vi "OCV Histogram gRPC.vi"() -> (1 "mean values of channels":dbl[](array[numeric]), 2 "std dev":dbl, 3 "range":dbl)   [LabVIEW 2019] (continued)
  out "Waveform Chart ch0":sgl[](graph)=[3.4816353, 3.4816356, 3.4816363, 3.4816382, 3.4816408, 3.48164, 3.481639, 3.4816341, 3.481641, 3.4816356, 3.4816346, 3.4816375, 3.4816372, 3.481637, 3.4816399, 3.4816375, 3.4816432, 3.4816358, 3.4816375, 3.48164, 3.4816394, 3.4816341, 3.4816387, 3.4816349, 3.4816382, 3.481638, 3.4816375, 3.4816344, 3.4816382, 3.4816399, 3.4816442, 3.4816413, 3.481636, 3.4816372, 3.4816327, 3.4816341, 3.4816403, 3.4816394, 3.4816413, 3.4816415, 3.4816406, 3.481637, 3.4816372, 3.4816396, 3.4816391, 3.481643, 3.4816375, 3.4816341, 3.4816446, 3.4816337, 3.4816325, 3.4816356, 3.4816365, 3.4816322, 3.4816391, 3.481637, 3.4816382, 3.4816358, 3.4816394, 3.481634, 3.4816377, 3.481638, 3.4816375, 3.4816403, 3.4816413, 3.4816382, 3.481636, 3.4816418, 3.4816382, 3.4816322, 3.4816375, 3.4816356, 3.481642, 3.4816384, 3.4816382, 3.4816365, 3.481637, 3.4816353, 3.4816394, 3.4816382, 3.4816437, 3.4816415, 3.4816375, 3.4816375, 3.4816418, 3.4816406, 3.4816408, 3.4816415, 3.4816391, 3.4816394, 3.4816334, 3.48164, 3.4816394, 3.481636, 3.4816372, 3.4816384, 3.4816353, 3.4816396, 3.4816408, 3.481637, 3.4816346, 3.4816408, 3.4816375, 3.4816356, 3.481638, 3.4816396, 3.4816358, 3.4816408, 3.4816396, 3.4816313, 3.481634, 3.4816365, 3.481638, 3.4816403, 3.4816394, 3.4816377, 3.4816372, 3.4816365, 3.4816365, 3.4816382, 3.481635, 3.481638, 3.481636, 3.4816415, 3.481636, 3.4816332, 3.4816341, 3.4816382, 3.4816413, 3.4816377, 3.4816337, 3.4816344, 3.4816356, 3.4816418, 3.4816408, 3.4816337, 3.4816363, 3.481636, 3.481641, 3.4816375, 3.4816408, 3.4816346, 3.4816341, 3.4816403, 3.4816408, 3.4816437, 3.4816349, 3.481637, 3.4816344, 3.481637, 3.4816344, 3.4816406, 3.4816418, 3.481639, 3.481636, 3.4816332, 3.481638, 3.4816372, 3.481633, 3.4816353, 3.4816415, 3.4816365, 3.481645, 3.4816349, 3.481638, 3.4816444, 3.481642, 3.4816356, 3.481642, 3.4816377, 3.4816396, 3.4816408, 3.4816327, 3.4816408, 3.4816368, 3.481637, 3.4816332, 3.481636, 3.481638, 3.4816399, 3.4816365, 3.4816375, 3.4816287, 3.481641, 3.4816341, 3.4816413, 3.4816396, 3.4816425, 3.4816406, 3.481635, 3.4816413, 3.4816387, 3.4816396, 3.4816391, 3.4816377, 3.4816406, 3.481641, 3.4816406, 3.481635, 3.4816337]
  out "Waveform Chart ch3":sgl[](graph)=[3.482367, 3.4823706, 3.4823644, 3.4823663, 3.48237, 3.4823658, 3.482369, 3.4823651, 3.482372, 3.4823728, 3.4823637, 3.4823651, 3.4823728, 3.482369, 3.4823713, 3.4823675, 3.482368, 3.4823685, 3.4823701, 3.4823718, 3.4823713, 3.4823737, 3.482368, 3.482367, 3.4823716, 3.4823666, 3.482369, 3.4823692, 3.4823682, 3.482368, 3.482372, 3.482368, 3.482369, 3.4823658, 3.48237, 3.4823718, 3.482369, 3.4823678, 3.482369, 3.4823713, 3.4823692, 3.4823666, 3.4823666, 3.4823713, 3.482368, 3.482366, 3.482367, 3.48237, 3.4823694, 3.4823694, 3.4823673, 3.482366, 3.4823682, 3.4823666, 3.4823685, 3.482366, 3.48237, 3.4823682, 3.4823692, 3.4823651, 3.482369, 3.48237, 3.4823647, 3.4823694, 3.482367, 3.4823701, 3.482367, 3.482368, 3.4823678, 3.4823651, 3.4823635, 3.482366, 3.482366, 3.4823685, 3.4823694, 3.4823656, 3.4823709, 3.4823658, 3.4823673, 3.4823682, 3.4823694, 3.482367, 3.482367, 3.4823663, 3.4823596, 3.4823644, 3.4823697, 3.4823694, 3.482368, 3.4823668, 3.4823647, 3.4823644, 3.482364, 3.4823663, 3.4823635, 3.4823613, 3.482367, 3.4823625, 3.4823687, 3.482369, 3.4823632, 3.4823682, 3.4823718, 3.4823654, 3.48237, 3.482371, 3.4823675, 3.4823616, 3.4823694, 3.482364, 3.4823709, 3.4823658, 3.4823692, 3.4823651, 3.4823654, 3.4823618, 3.4823678, 3.4823644, 3.4823694, 3.4823668, 3.482365, 3.4823606, 3.4823675, 3.4823725, 3.4823642, 3.4823651, 3.4823678, 3.4823651, 3.4823666, 3.4823637, 3.4823608, 3.4823682, 3.4823635, 3.4823654, 3.4823651, 3.4823635, 3.482366, 3.482362, 3.4823654, 3.4823697, 3.4823678, 3.482368, 3.4823656, 3.4823704, 3.4823687, 3.482368, 3.4823687, 3.4823644, 3.4823673, 3.4823682, 3.48237, 3.4823701, 3.4823663, 3.4823632, 3.482362, 3.4823678, 3.4823663, 3.482365, 3.4823642, 3.4823697, 3.4823642, 3.4823658, 3.4823675, 3.482364, 3.4823694, 3.4823692, 3.482372, 3.482364, 3.4823654, 3.4823654, 3.4823637, 3.482367, 3.4823623, 3.482365, 3.4823625, 3.4823656, 3.482365, 3.4823658, 3.4823635, 3.4823668, 3.4823666, 3.482368, 3.4823678, 3.482362, 3.4823651, 3.4823654, 3.4823692, 3.4823673, 3.4823668, 3.4823666, 3.482364, 3.4823673, 3.4823701, 3.4823651, 3.4823647, 3.4823635, 3.4823675, 3.4823632, 3.4823704, 3.4823666]
  out "Results Cluster":T4={"Waveform Chart ch0"=[3.481635332107544, 3.481635570526123, 3.4816362857818604, 3.481638193130493, 3.4816408157348633, 3.481640100479126, 3.4816389083862305, 3.4816341400146484, 3.4816410541534424, 3.481635570526123, 3.4816346168518066, 3.481637477874756, 3.4816372394561768, 3.4816370010375977, 3.481639862060547, 3.481637477874756, 3.4816431999206543, 3.481635808944702, 3.481637477874756, 3.481640100479126, 3.4816393852233887, 3.4816341400146484, 3.4816386699676514, 3.4816348552703857, 3.481638193130493, 3.481637954711914, 3.481637477874756, 3.4816343784332275, 3.481638193130493, 3.481639862060547, 3.4816441535949707, 3.4816412925720215, 3.4816360473632812, 3.4816372394561768, 3.481632709503174, 3.4816341400146484, 3.481640338897705, 3.4816393852233887, 3.4816412925720215, 3.4816415309906006, 3.481640577316284, 3.4816370010375977, 3.4816372394561768, 3.4816396236419678, 3.4816391468048096, 3.481642961502075, 3.481637477874756, 3.4816341400146484, 3.481644630432129, 3.4816336631774902, 3.4816324710845947, 3.481635570526123, 3.4816365242004395, 3.4816322326660156, 3.4816391468048096, 3.4816370010375977, 3.481638193130493, 3.481635808944702, 3.4816393852233887, 3.4816339015960693, 3.481637716293335, 3.481637954711914, 3.481637477874756, 3.481640338897705, 3.4816412925720215, 3.481638193130493, 3.4816360473632812, 3.4816417694091797, 3.481638193130493, 3.4816322326660156, 3.481637477874756, 3.481635570526123, 3.481642007827759, 3.4816384315490723, 3.481638193130493, 3.4816365242004395, 3.4816370010375977, 3.481635332107544, 3.4816393852233887, 3.481638193130493, 3.4816436767578125, 3.4816415309906006, 3.481637477874756, 3.481637477874756, 3.4816417694091797, 3.481640577316284, 3.4816408157348633, 3.4816415309906006, 3.4816391468048096, 3.4816393852233887, 3.481633424758911, 3.481640100479126, 3.4816393852233887, 3.4816360473632812, 3.4816372394561768, 3.4816384315490723, 3.481635332107544, 3.4816396236419678, 3.4816408157348633, 3.4816370010375977, 3.4816346168518066, 3.4816408157348633, 3.481637477874756, 3.481635570526123, 3.481637954711914, 3.4816396236419678, 3.481635808944702, 3.4816408157348633, 3.4816396236419678, 3.481631278991699, 3.4816339015960693, 3.4816365242004395, 3.481637954711914, 3.481640338897705, 3.4816393852233887, 3.481637716293335, 3.4816372394561768, 3.4816365242004395, 3.4816365242004395, 3.481638193130493, 3.481635093688965, 3.481637954711914, 3.4816360473632812, 3.4816415309906006, 3.4816360473632812, 3.481633186340332, 3.4816341400146484, 3.481638193130493, 3.4816412925720215, 3.481637716293335, 3.4816336631774902, 3.4816343784332275, 3.481635570526123, 3.4816417694091797, 3.4816408157348633, 3.4816336631774902, 3.4816362857818604, 3.4816360473632812, 3.4816410541534424, 3.481637477874756, 3.4816408157348633, 3.4816346168518066, 3.4816341400146484, 3.481640338897705, 3.4816408157348633, 3.4816436767578125, 3.4816348552703857, 3.4816370010375977, 3.4816343784332275, 3.4816370010375977, 3.4816343784332275, 3.481640577316284, 3.4816417694091797, 3.4816389083862305, 3.4816360473632812, 3.481633186340332, 3.481637954711914, 3.4816372394561768, 3.481632947921753, 3.481635332107544, 3.4816415309906006, 3.4816365242004395, 3.481645107269287, 3.4816348552703857, 3.481637954711914, 3.48164439201355, 3.481642007827759, 3.481635570526123, 3.481642007827759, 3.481637716293335, 3.4816396236419678, 3.4816408157348633, 3.481632709503174, 3.4816408157348633, 3.4816367626190186, 3.4816370010375977, 3.481633186340332, 3.4816360473632812, 3.481637954711914, 3.481639862060547, 3.4816365242004395, 3.481637477874756, 3.481628656387329, 3.4816410541534424, 3.4816341400146484, 3.4816412925720215, 3.4816396236419678, 3.481642484664917, 3.481640577316284, 3.481635093688965, 3.4816412925720215, 3.4816386699676514, 3.4816396236419678, 3.4816391468048096, 3.481637716293335, 3.481640577316284, 3.4816410541534424, 3.481640577316284, 3.481635093688965, 3.4816336631774902], "ch0 mean"=3.4816378843784332, "ch0 range"=1.6450881958007812e-05, "ch0 std dev"=2.907318571584298e-06, "Histogram Graph ch0"={"X Values"=[3.481629478931427, 3.4816311240196227, 3.4816327691078186, 3.4816344141960145, 3.4816360592842104, 3.4816377043724063, 3.481639349460602, 3.481640994548798, 3.481642639636994, 3.48164428472519], "Histogram: h(x)"=[1, 1, 10, 26, 32, 51, 28, 39, 6, 6]}, "Waveform Chart ch1"=[3.4830455780029297, 3.483036756515503, 3.4830386638641357, 3.483046770095825, 3.483046531677246, 3.4830381870269775, 3.483044385910034, 3.4830410480499268, 3.483041763305664, 3.483039617538452, 3.483038902282715, 3.4830398559570312, 3.483046293258667, 3.483041286468506, 3.4830386638641357, 3.4830422401428223, 3.4830386638641357, 3.4830429553985596, 3.4830410480499268, 3.483044385910034, 3.4830453395843506, 3.483041286468506, 3.4830446243286133, 3.4830400943756104, 3.4830410480499268, 3.4830427169799805, 3.483039617538452, 3.4830408096313477, 3.4830451011657715, 3.4830451011657715, 3.483037233352661, 3.483043670654297, 3.483041763305664, 3.4830408096313477, 3.4830405712127686, 3.4830384254455566, 3.483039379119873, 3.4830453395843506, 3.483045816421509, 3.483043670654297, 3.4830434322357178, 3.4830405712127686, 3.4830427169799805, 3.483043909072876, 3.4830427169799805, 3.4830446243286133, 3.4830431938171387, 3.483044385910034, 3.4830422401428223, 3.483038902282715, 3.483041286468506, 3.483046054840088, 3.483045816421509, 3.483044385910034, 3.483041286468506, 3.4830398559570312, 3.4830427169799805, 3.4830434322357178, 3.483043909072876, 3.4830408096313477, 3.4830424785614014, 3.483038902282715, 3.4830474853515625, 3.4830472469329834, 3.4830482006073, 3.4830446243286133, 3.4830408096313477, 3.483041763305664, 3.483042001724243, 3.4830374717712402, 3.4830381870269775, 3.483039140701294, 3.483043909072876, 3.4830429553985596, 3.4830403327941895, 3.4830384254455566, 3.483041286468506, 3.4830470085144043, 3.483037233352661, 3.4830408096313477, 3.483042001724243, 3.483048915863037, 3.483037233352661, 3.4830410480499268, 3.483036756515503, 3.483046293258667, 3.4830424785614014, 3.4830429553985596, 3.483044147491455, 3.483039140701294, 3.4830398559570312, 3.4830377101898193, 3.483043670654297, 3.4830400943756104, 3.483039379119873, 3.4830451011657715, 3.483041763305664, 3.4830474853515625, 3.483044147491455, 3.4830446243286133, 3.4830362796783447, 3.4830429553985596, 3.483043909072876, 3.4830429553985596, 3.483041763305664, 3.483039140701294, 3.4830422401428223, 3.4830386638641357, 3.483044385910034, 3.4830422401428223, 3.483035087585449, 3.4830429553985596, 3.4830424785614014, 3.483042001724243, 3.483042001724243, 3.4830355644226074, 3.483041286468506, 3.4830424785614014, 3.483042001724243, 3.483044147491455, 3.483039140701294, 3.4830470085144043, 3.483041524887085, 3.4830403327941895, 3.4830405712127686, 3.483046531677246, 3.483044385910034, 3.4830379486083984, 3.483039617538452, 3.483036994934082, 3.483041763305664, 3.483046054840088, 3.483043909072876, 3.4830455780029297, 3.4830448627471924, 3.4830386638641357, 3.4830429553985596, 3.483048439025879, 3.4830405712127686, 3.4830455780029297, 3.4830403327941895, 3.483043909072876, 3.4830408096313477, 3.483039379119873, 3.4830410480499268, 3.4830434322357178, 3.483044147491455, 3.4830405712127686, 3.4830405712127686, 3.483046770095825, 3.4830429553985596, 3.4830477237701416, 3.483041524887085, 3.483043909072876, 3.483039617538452, 3.4830451011657715, 3.483045816421509, 3.4830472469329834, 3.483039379119873, 3.4830424785614014, 3.4830448627471924, 3.4830422401428223, 3.483045816421509, 3.4830405712127686, 3.483042001724243, 3.4830453395843506, 3.483048915863037, 3.4830408096313477, 3.4830410480499268, 3.4830405712127686, 3.483045816421509, 3.48305082321167, 3.4830398559570312, 3.483038902282715, 3.483042001724243, 3.483041763305664, 3.4830405712127686, 3.483038902282715, 3.483045816421509, 3.4830424785614014, 3.483036518096924, 3.4830470085144043, 3.483041763305664, 3.4830431938171387, 3.483041524887085, 3.483046054840088, 3.4830405712127686, 3.483041763305664, 3.483046293258667, 3.4830434322357178, 3.483041524887085, 3.4830422401428223, 3.483043670654297, 3.483041286468506, 3.4830374717712402, 3.4830424785614014, 3.4830472469329834, 3.4830381870269775, 3.483037233352661, 3.4830379486083984], "ch1 mean"=3.4830422377586365, "ch1 range"=1.5735626220703125e-05, "ch1 std dev"=2.9857574743435946e-06, "Histogram Graph ch1"={"X Values"=[3.4830358743667604, 3.4830374479293824, 3.4830390214920044, 3.4830405950546264, 3.4830421686172484, 3.4830437421798703, 3.4830453157424923, 3.4830468893051143, 3.4830484628677363, 3.4830500364303583], "Histogram: h(x)"=[4, 15, 24, 39, 37, 35, 25, 15, 5, 1]}, "Waveform Chart ch2"=[3.4783694744110107, 3.4783682823181152, 3.4783730506896973, 3.478372097015381, 3.4783780574798584, 3.478374719619751, 3.47836971282959, 3.478370428085327, 3.4783718585968018, 3.4783709049224854, 3.4783730506896973, 3.4783737659454346, 3.478377103805542, 3.478372812271118, 3.478370189666748, 3.4783687591552734, 3.4783730506896973, 3.4783685207366943, 3.4783713817596436, 3.47836971282959, 3.47837233543396, 3.478372812271118, 3.4783685207366943, 3.478372812271118, 3.4783732891082764, 3.478370428085327, 3.4783682823181152, 3.478372812271118, 3.4783670902252197, 3.4783711433410645, 3.4783737659454346, 3.478374719619751, 3.4783737659454346, 3.4783713817596436, 3.478369951248169, 3.478365182876587, 3.4783737659454346, 3.478370189666748, 3.478368043899536, 3.478376626968384, 3.478376626968384, 3.4783709049224854, 3.47836971282959, 3.478375196456909, 3.4783709049224854, 3.4783756732940674, 3.478369951248169, 3.478367805480957, 3.47837233543396, 3.4783668518066406, 3.478365182876587, 3.478368043899536, 3.478370189666748, 3.478375196456909, 3.478372812271118, 3.478374481201172, 3.47836971282959, 3.4783742427825928, 3.4783754348754883, 3.4783668518066406, 3.4783716201782227, 3.478365421295166, 3.4783782958984375, 3.47837233543396, 3.4783694744110107, 3.4783735275268555, 3.4783682823181152, 3.4783668518066406, 3.47837233543396, 3.4783689975738525, 3.4783709049224854, 3.4783694744110107, 3.4783706665039062, 3.478372812271118, 3.4783694744110107, 3.4783713817596436, 3.478368043899536, 3.4783692359924316, 3.478367805480957, 3.4783668518066406, 3.478370428085327, 3.478370189666748, 3.4783694744110107, 3.4783754348754883, 3.4783687591552734, 3.47836971282959, 3.478372812271118, 3.4783737659454346, 3.4783682823181152, 3.4783737659454346, 3.4783709049224854, 3.4783706665039062, 3.478374481201172, 3.4783668518066406, 3.4783740043640137, 3.478372812271118, 3.478372812271118, 3.4783694744110107, 3.4783737659454346, 3.4783685207366943, 3.478369951248169, 3.478376626968384, 3.4783730506896973, 3.478367805480957, 3.4783711433410645, 3.4783670902252197, 3.478368043899536, 3.478365421295166, 3.4783780574798584, 3.4783711433410645, 3.4783713817596436, 3.478365898132324, 3.4783754348754883, 3.478374481201172, 3.4783716201782227, 3.4783716201782227, 3.4783735275268555, 3.478370428085327, 3.4783668518066406, 3.4783742427825928, 3.478374481201172, 3.478372097015381, 3.478374719619751, 3.478372812271118, 3.47836971282959, 3.4783716201782227, 3.4783694744110107, 3.4783670902252197, 3.478374719619751, 3.47837233543396, 3.4783666133880615, 3.4783737659454346, 3.4783732891082764, 3.4783713817596436, 3.4783735275268555, 3.4783740043640137, 3.4783644676208496, 3.4783742427825928, 3.4783663749694824, 3.4783711433410645, 3.478377103805542, 3.4783706665039062, 3.4783692359924316, 3.478372097015381, 3.4783754348754883, 3.4783713817596436, 3.4783682823181152, 3.4783692359924316, 3.4783663749694824, 3.478372812271118, 3.4783687591552734, 3.4783761501312256, 3.4783730506896973, 3.4783706665039062, 3.4783642292022705, 3.4783718585968018, 3.4783735275268555, 3.4783737659454346, 3.4783713817596436, 3.4783754348754883, 3.478379249572754, 3.4783711433410645, 3.4783716201782227, 3.478369951248169, 3.4783694744110107, 3.4783740043640137, 3.4783735275268555, 3.4783732891082764, 3.4783692359924316, 3.478376626968384, 3.4783735275268555, 3.4783718585968018, 3.4783666133880615, 3.478365421295166, 3.4783709049224854, 3.478372573852539, 3.4783666133880615, 3.4783718585968018, 3.4783742427825928, 3.478364944458008, 3.478368043899536, 3.478372812271118, 3.47836971282959, 3.478370189666748, 3.47837495803833, 3.4783718585968018, 3.4783689975738525, 3.47836971282959, 3.4783732891082764, 3.4783709049224854, 3.4783785343170166, 3.478369951248169, 3.4783735275268555, 3.478372573852539, 3.4783682823181152, 3.47836971282959, 3.4783763885498047, 3.4783670902252197, 3.478369951248169, 3.478370189666748], "ch2 mean"=3.478371295928955, "ch2 range"=1.5020370483398438e-05, "ch2 std dev"=3.0624530062047095e-06, "Histogram Graph ch2"={"X Values"=[3.4783649802207948, 3.4783664822578433, 3.478367984294892, 3.4783694863319403, 3.478370988368989, 3.4783724904060374, 3.478373992443086, 3.4783754944801344, 3.478376996517183, 3.4783784985542314], "Histogram: h(x)"=[8, 16, 17, 38, 32, 32, 35, 10, 7, 5]}, "Waveform Chart ch3"=[3.4823670387268066, 3.482370615005493, 3.4823644161224365, 3.4823663234710693, 3.482369899749756, 3.482365846633911, 3.4823689460754395, 3.482365131378174, 3.4823720455169678, 3.482372760772705, 3.482363700866699, 3.482365131378174, 3.482372760772705, 3.4823689460754395, 3.4823713302612305, 3.482367515563965, 3.482367992401123, 3.4823684692382812, 3.482370138168335, 3.4823718070983887, 3.4823713302612305, 3.4823737144470215, 3.482367992401123, 3.4823670387268066, 3.4823715686798096, 3.4823665618896484, 3.4823689460754395, 3.4823691844940186, 3.482368230819702, 3.482367992401123, 3.4823720455169678, 3.482367992401123, 3.4823689460754395, 3.482365846633911, 3.482369899749756, 3.4823718070983887, 3.4823689460754395, 3.482367753982544, 3.4823689460754395, 3.4823713302612305, 3.4823691844940186, 3.4823665618896484, 3.4823665618896484, 3.4823713302612305, 3.482367992401123, 3.4823660850524902, 3.4823670387268066, 3.482369899749756, 3.4823694229125977, 3.4823694229125977, 3.4823672771453857, 3.4823660850524902, 3.482368230819702, 3.4823665618896484, 3.4823684692382812, 3.4823660850524902, 3.482369899749756, 3.482368230819702, 3.4823691844940186, 3.482365131378174, 3.4823689460754395, 3.482369899749756, 3.4823646545410156, 3.4823694229125977, 3.4823670387268066, 3.482370138168335, 3.4823670387268066, 3.482367992401123, 3.482367753982544, 3.482365131378174, 3.48236346244812, 3.4823660850524902, 3.4823660850524902, 3.4823684692382812, 3.4823694229125977, 3.482365608215332, 3.4823708534240723, 3.482365846633911, 3.4823672771453857, 3.482368230819702, 3.4823694229125977, 3.4823670387268066, 3.4823670387268066, 3.4823663234710693, 3.4823596477508545, 3.4823644161224365, 3.4823696613311768, 3.4823694229125977, 3.482367992401123, 3.4823668003082275, 3.4823646545410156, 3.4823644161224365, 3.4823639392852783, 3.4823663234710693, 3.48236346244812, 3.482361316680908, 3.4823670387268066, 3.4823625087738037, 3.4823687076568604, 3.4823689460754395, 3.482363224029541, 3.482368230819702, 3.4823718070983887, 3.482365369796753, 3.482369899749756, 3.4823710918426514, 3.482367515563965, 3.4823615550994873, 3.4823694229125977, 3.4823639392852783, 3.4823708534240723, 3.482365846633911, 3.4823691844940186, 3.482365131378174, 3.482365369796753, 3.4823617935180664, 3.482367753982544, 3.4823644161224365, 3.4823694229125977, 3.4823668003082275, 3.4823648929595947, 3.482360601425171, 3.482367515563965, 3.482372522354126, 3.4823641777038574, 3.482365131378174, 3.482367753982544, 3.482365131378174, 3.4823665618896484, 3.482363700866699, 3.48236083984375, 3.482368230819702, 3.48236346244812, 3.482365369796753, 3.482365131378174, 3.48236346244812, 3.4823660850524902, 3.4823620319366455, 3.482365369796753, 3.4823696613311768, 3.482367753982544, 3.482367992401123, 3.482365608215332, 3.482370376586914, 3.4823687076568604, 3.482367992401123, 3.4823687076568604, 3.4823644161224365, 3.4823672771453857, 3.482368230819702, 3.482369899749756, 3.482370138168335, 3.4823663234710693, 3.482363224029541, 3.4823620319366455, 3.482367753982544, 3.4823663234710693, 3.4823648929595947, 3.4823641777038574, 3.4823696613311768, 3.4823641777038574, 3.482365846633911, 3.482367515563965, 3.4823639392852783, 3.4823694229125977, 3.4823691844940186, 3.4823720455169678, 3.4823639392852783, 3.482365369796753, 3.482365369796753, 3.482363700866699, 3.4823670387268066, 3.4823622703552246, 3.4823648929595947, 3.4823625087738037, 3.482365608215332, 3.4823648929595947, 3.482365846633911, 3.48236346244812, 3.4823668003082275, 3.4823665618896484, 3.482367992401123, 3.482367753982544, 3.4823620319366455, 3.482365131378174, 3.482365369796753, 3.4823691844940186, 3.4823672771453857, 3.4823668003082275, 3.4823665618896484, 3.4823639392852783, 3.4823672771453857, 3.482370138168335, 3.482365131378174, 3.4823646545410156, 3.48236346244812, 3.482367515563965, 3.482363224029541, 3.482370376586914, 3.4823665618896484], "ch3 mean"=3.4823670625686645, "ch3 range"=1.4066696166992188e-05, "ch3 std dev"=2.703397559171438e-06, "Histogram Graph ch3"={"X Values"=[3.4823603510856627, 3.4823617577552795, 3.4823631644248962, 3.482364571094513, 3.48236597776413, 3.4823673844337466, 3.4823687911033634, 3.48237019777298, 3.482371604442597, 3.4823730111122138], "Histogram: h(x)"=[3, 7, 14, 30, 35, 40, 36, 19, 12, 4]}, "Waveform Chart ch4"=[3.4843995571136475, 3.484405755996704, 3.484407663345337, 3.484403610229492, 3.48439884185791, 3.4843997955322266, 3.484405755996704, 3.4844071865081787, 3.484409809112549, 3.484401226043701, 3.4844048023223877, 3.4844062328338623, 3.4844040870666504, 3.484405040740967, 3.484408378601074, 3.4843993186950684, 3.484402894973755, 3.484402894973755, 3.484405040740967, 3.484403133392334, 3.484398365020752, 3.4844045639038086, 3.4844067096710205, 3.4844062328338623, 3.484405279159546, 3.4844048023223877, 3.484407663345337, 3.4844024181365967, 3.4844069480895996, 3.4843976497650146, 3.484405279159546, 3.484398365020752, 3.4844093322753906, 3.4844064712524414, 3.484407424926758, 3.484405279159546, 3.4843952655792236, 3.4844062328338623, 3.484409809112549, 3.484401226043701, 3.4844048023223877, 3.4844093322753906, 3.4844093322753906, 3.484403610229492, 3.4844048023223877, 3.48439884185791, 3.4844114780426025, 3.4844045639038086, 3.4844014644622803, 3.4844107627868652, 3.4844014644622803, 3.4844064712524414, 3.484400987625122, 3.4844021797180176, 3.484400510787964, 3.4844045639038086, 3.4844014644622803, 3.4844017028808594, 3.484400510787964, 3.4844038486480713, 3.484400987625122, 3.4844064712524414, 3.4844038486480713, 3.4843976497650146, 3.4844043254852295, 3.48439621925354, 3.484405994415283, 3.4844110012054443, 3.484405279159546, 3.484405040740967, 3.4844062328338623, 3.484405755996704, 3.484402656555176, 3.484408140182495, 3.4844038486480713, 3.484405994415283, 3.4844017028808594, 3.4844014644622803, 3.484403371810913, 3.4844112396240234, 3.4844021797180176, 3.484403371810913, 3.484405279159546, 3.4843974113464355, 3.484407901763916, 3.4843990802764893, 3.4844019412994385, 3.484398603439331, 3.48439884185791, 3.484403371810913, 3.484400749206543, 3.484405994415283, 3.4843995571136475, 3.4844069480895996, 3.484405755996704, 3.484400749206543, 3.484400510787964, 3.4844000339508057, 3.4844045639038086, 3.484408140182495, 3.484402656555176, 3.484398603439331, 3.4844017028808594, 3.484403610229492, 3.4843993186950684, 3.4844043254852295, 3.4844017028808594, 3.4844038486480713, 3.4844000339508057, 3.484405755996704, 3.4844048023223877, 3.4844069480895996, 3.4844002723693848, 3.4844043254852295, 3.484403133392334, 3.484405040740967, 3.4844071865081787, 3.484407901763916, 3.484405755996704, 3.484402656555176, 3.48439884185791, 3.4844024181365967, 3.4844071865081787, 3.4844048023223877, 3.484403133392334, 3.4843995571136475, 3.4844014644622803, 3.4843995571136475, 3.484405279159546, 3.484405279159546, 3.484405040740967, 3.484400510787964, 3.4844043254852295, 3.4844021797180176, 3.4844014644622803, 3.484405994415283, 3.4844090938568115, 3.4843971729278564, 3.4843993186950684, 3.4843976497650146, 3.484400987625122, 3.484405040740967, 3.484400510787964, 3.4844024181365967, 3.4843971729278564, 3.4844014644622803, 3.4844038486480713, 3.484398603439331, 3.484400749206543, 3.4843997955322266, 3.484405755996704, 3.4844017028808594, 3.4843976497650146, 3.484398603439331, 3.4844024181365967, 3.484403133392334, 3.48439884185791, 3.4843976497650146, 3.4843976497650146, 3.4844024181365967, 3.4843974113464355, 3.4844017028808594, 3.4844000339508057, 3.484405517578125, 3.4844021797180176, 3.48439884185791, 3.48439621925354, 3.4844062328338623, 3.4843974113464355, 3.4843990802764893, 3.4843974113464355, 3.484395980834961, 3.4844002723693848, 3.484407424926758, 3.484403371810913, 3.484400987625122, 3.484405755996704, 3.484405517578125, 3.484398365020752, 3.484395742416382, 3.4844019412994385, 3.4843995571136475, 3.484405040740967, 3.484400987625122, 3.4844014644622803, 3.4843997955322266, 3.4844040870666504, 3.484403133392334, 3.484401226043701, 3.484402894973755, 3.4843997955322266, 3.484403371810913, 3.4843990802764893, 3.4844019412994385, 3.4844048023223877, 3.484402894973755, 3.484405994415283, 3.4844095706939697, 3.4844069480895996, 3.4844045639038086], "ch4 mean"=3.4844029903411866, "ch4 range"=1.621246337890625e-05, "ch4 std dev"=3.4826254869466815e-06, "Histogram Graph ch4"={"X Values"=[3.4843960762023927, 3.4843976974487307, 3.484399318695069, 3.484400939941407, 3.484402561187745, 3.484404182434083, 3.484405803680421, 3.484407424926759, 3.484409046173097, 3.4844106674194353], "Histogram: h(x)"=[5, 15, 28, 32, 24, 31, 37, 16, 8, 4]}} {"ch4 range" format="%#_6p"; "ch4 std dev" format="%#.3p"; "ch4 mean" format="%#.6p"; "ch3 range" format="%#_6p"; "ch3 std dev" format="%#.3p"; "ch3 mean" format="%#.6p"; "ch2 range" format="%#_6p"; "ch2 std dev" format="%#.3p"; "ch2 mean" format="%#.6p"; "ch1 range" format="%#_6p"; "ch1 std dev" format="%#.3p"; "ch1 mean" format="%#.6p"; "ch0 range" format="%#_6p"; "ch0 std dev" format="%#.3p"; "ch0 mean" format="%#.6p"}
  in  "Results Cluster":T4={"Waveform Chart ch0"=[-6.482741875349764e-06, -6.609674165618734e-06, -6.233203080218623e-06, -6.613210951394088e-06, -5.909245924550351e-06, -6.1328996888307884e-06, -6.358200673203053e-06, -6.870973185430456e-06, -6.243427483099904e-06, -5.953840097279857e-06, -6.577614794730629e-06, -5.768388563769013e-06, -5.889962020259323e-06, -5.91212430154465e-06, -6.419565311385181e-06, -6.50829315132552e-06, -5.536830131867864e-06, -6.271011369459595e-06, -6.937542782195293e-06, -7.44168991871554e-06, -6.8984467501811205e-06, -7.4441074466820366e-06, -6.884514522294152e-06, -7.229455884586274e-06, -7.204633996616539e-06, -7.520671633596594e-06, -7.348344858091178e-06, -7.026224856705287e-06, -6.4957495291395714e-06, -6.9697185324009035e-06, -6.64170832689038e-06, -6.516226556717238e-06, -6.80187883727134e-06, -7.473746530800666e-06, -6.8019074543289836e-06, -6.421730747707948e-06, -6.915517716049444e-06, -7.233306065769019e-06, -6.9335647318597554e-06, -6.495809932905111e-06], "ch0 mean"=-6.648192609520545e-06, "ch0 range"=1.9838415017287296e-06, "ch0 std dev"=5.022029434534627e-07, "Histogram Graph ch0"={"X Values"=[-7.4214795585101575e-06, -7.223095408337285e-06, -7.024711258164412e-06, -6.82632710799154e-06, -6.627942957818667e-06, -6.4295588076457944e-06, -6.231174657472922e-06, -6.032790507300049e-06, -5.8344063571271766e-06, -5.636022206954304e-06], "Histogram: h(x)"=[5, 3, 4, 6, 4, 8, 4, 1, 4, 1]}, "Waveform Chart ch1"=[-2.622437675041801e-06, -2.1054414953660847e-06, -2.3277676624794484e-06, -2.558376653803712e-06, -2.2236999675494533e-06, -2.589016451053761e-06, -2.6354278960691e-06, -2.7367192087189563e-06, -2.424017879995447e-06, -3.0489161443253215e-06, -3.1442148467963687e-06, -2.4032855210096374e-06, -2.569647882839888e-06, -2.4698150005498013e-06, -3.0781658817195746e-06, -2.377010372332436e-06, -2.0435595699758798e-06, -2.106839167327596e-06, -1.7412107178156014e-06, -3.2480049993772076e-06, -1.9805074376907754e-06, -2.5608807141114243e-06, -2.18054640635336e-06, -3.099457174386434e-06, -3.102303246629032e-06, -3.2920758007788295e-06, -3.3778499352142414e-06, -3.3187560901861313e-06, -3.484840052811922e-06, -3.485501008160019e-06, -2.8728971850629594e-06, -2.6623123946996634e-06, -2.187546597757112e-06, -2.5467930720162336e-06, -2.7862697099761513e-06, -2.528638777412977e-06, -2.0537236385737207e-06, -2.5329982714180255e-06, -2.7424337661967574e-06, -3.067742416854491e-06], "ch1 mean"=-2.6579412172609335e-06, "ch1 range"=1.7442902903444177e-06, "ch1 std dev"=4.468204660544414e-07, "Histogram Graph ch1"={"X Values"=[-3.3982864936427982e-06, -3.2238574646083565e-06, -3.0494284355739147e-06, -2.874999406539473e-06, -2.700570377505031e-06, -2.5261413484705894e-06, -2.3517123194361476e-06, -2.177283290401706e-06, -2.002854261367264e-06, -1.8284252323328223e-06], "Histogram: h(x)"=[4, 3, 5, 1, 6, 8, 4, 5, 3, 1]}, "Waveform Chart ch2"=[5.544446756924017e-06, 5.893818847440082e-06, 5.6959361744068e-06, 6.353655436755351e-06, 6.650659273380882e-06, 6.187390686867271e-06, 6.20360970192913e-06, 5.7770612172558695e-06, 5.816303483036932e-06, 5.681492261411933e-06, 5.92762437831725e-06, 6.190843181120228e-06, 5.928079790707314e-06, 6.068116911256402e-06, 6.161619546592655e-06, 5.5543262999422065e-06, 6.17040032539053e-06, 5.4655577958543896e-06, 5.76704970728763e-06, 6.0194055222271105e-06, 5.783390336812049e-06, 5.768011867723238e-06, 6.0153044120154e-06, 6.001437704705948e-06, 5.911709913790112e-06, 5.830095407868431e-06, 5.25398022881523e-06, 5.15697143423068e-06, 4.826305970962092e-06, 5.462550730311096e-06, 5.059430867978049e-06, 5.682513029845579e-06, 5.851683523904261e-06, 5.099226732675129e-06, 5.2309820281174504e-06, 5.22374278950658e-06, 5.829274618675769e-06, 4.746499851558932e-06, 5.396447289671177e-06, 6.039472630669777e-06], "ch2 mean"=5.730660716698524e-06, "ch2 range"=1.9041594218219493e-06, "ch2 std dev"=4.1579103732429095e-07, "Histogram Graph ch2"={"X Values"=[4.8417078226500296e-06, 5.032123764832224e-06, 5.222539707014419e-06, 5.412955649196613e-06, 5.603371591378808e-06, 5.7937875335610025e-06, 5.984203475743197e-06, 6.174619417925392e-06, 6.365035360107586e-06, 6.555451302289781e-06], "Histogram: h(x)"=[2, 2, 4, 3, 5, 8, 9, 5, 1, 1]}, "Waveform Chart ch3"=[9.329772359568193e-06, 9.772186603754015e-06, 9.974785258468733e-06, 1.02561315552989e-05, 9.495402230894659e-06, 9.736598828932665e-06, 9.898850155608759e-06, 1.0197036488504313e-05, 9.305987891150035e-06, 9.316802834906767e-06, 9.746712874470878e-06, 9.737416581604666e-06, 9.867514527065477e-06, 9.509080464808271e-06, 9.481845866845764e-06, 9.70755176396829e-06, 8.885838770613302e-06, 9.475699672125386e-06, 9.258180372816345e-06, 9.834891872602234e-06, 9.402243918552161e-06, 9.713205786936326e-06, 9.876491292911543e-06, 9.871789580104262e-06, 9.650930388911628e-06, 9.41118365911455e-06, 9.575353492249282e-06, 9.196921234035763e-06, 9.15123272945548e-06, 8.949563027841687e-06, 9.474861956745276e-06, 8.825224921180636e-06, 8.727701114334558e-06, 9.16860173648142e-06, 8.905227736485157e-06, 9.144446889757383e-06, 8.885482293855075e-06, 9.859395612279415e-06, 9.32444154185109e-06, 9.310827508550253e-06], "ch3 mean"=9.480335334891014e-06, "ch3 range"=1.5284304409643419e-06, "ch3 std dev"=3.7432297421944963e-07, "Histogram Graph ch3"={"X Values"=[8.804122636382775e-06, 8.956965680479209e-06, 9.109808724575643e-06, 9.262651768672077e-06, 9.415494812768511e-06, 9.568337856864946e-06, 9.72118090096138e-06, 9.874023945057814e-06, 1.0026866989154248e-05, 1.0179710033250682e-05], "Histogram: h(x)"=[2, 4, 3, 7, 5, 3, 7, 6, 1, 2]}, "Waveform Chart ch4"=[9.329772359568193e-06, 9.772186603754015e-06, 9.974785258468733e-06, 1.02561315552989e-05, 9.495402230894659e-06, 9.736598828932665e-06, 9.898850155608759e-06, 1.0197036488504313e-05, 9.305987891150035e-06, 9.316802834906767e-06, 9.746712874470878e-06, 9.737416581604666e-06, 9.867514527065477e-06, 9.509080464808271e-06, 9.481845866845764e-06, 9.70755176396829e-06, 8.885838770613302e-06, 9.475699672125386e-06, 9.258180372816345e-06, 9.834891872602234e-06, 9.402243918552161e-06, 9.713205786936326e-06, 9.876491292911543e-06, 9.871789580104262e-06, 9.650930388911628e-06, 9.41118365911455e-06, 9.575353492249282e-06, 9.196921234035763e-06, 9.15123272945548e-06, 8.949563027841687e-06, 9.474861956745276e-06, 8.825224921180636e-06, 8.727701114334558e-06, 9.16860173648142e-06, 8.905227736485157e-06, 9.144446889757383e-06, 8.885482293855075e-06, 9.859395612279415e-06, 9.32444154185109e-06, 9.310827508550253e-06], "ch4 mean"=9.480335334891014e-06, "ch4 range"=1.5284304409643419e-06, "ch4 std dev"=3.7432297421944963e-07, "Histogram Graph ch4"={"X Values"=[8.804122636382775e-06, 8.956965680479209e-06, 9.109808724575643e-06, 9.262651768672077e-06, 9.415494812768511e-06, 9.568337856864946e-06, 9.72118090096138e-06, 9.874023945057814e-06, 1.0026866989154248e-05, 1.0179710033250682e-05], "Histogram: h(x)"=[2, 4, 3, 7, 5, 3, 7, 6, 1, 2]}} {"ch4 range" format="%#_6p"; "ch4 std dev" format="%#.3p"; "ch4 mean" format="%#.6p"; "ch3 range" format="%#_6p"; "ch3 std dev" format="%#.3p"; "ch3 mean" format="%#.6p"; "ch2 range" format="%#_6p"; "ch2 std dev" format="%#.3p"; "ch2 mean" format="%#.6p"; "ch1 range" format="%#_6p"; "ch1 std dev" format="%#.3p"; "ch1 mean" format="%#.6p"; "ch0 range" format="%#_6p"; "ch0 std dev" format="%#.3p"; "ch0 mean" format="%#.6p"}
  in  "OCVResults 1kHz":T1[](array[typedef])=[{"battery1voltage"=3.4816353, "battery2voltage"=3.4830456, "battery3voltage"=3.4783695, "battery4voltage"=3.482367, "battery5voltage"=3.4843996, "battery6voltage"=0.0, "battery7voltage"=0.0, "battery8voltage"=0.0, "battery9voltage"=0.0, "battery10voltage"=0.0, "battery11voltage"=0.0, "battery12voltage"=0.0, "battery13voltage"=0.0, "battery14voltage"=0.0, "battery15voltage"=0.0, "battery16voltage"=0.0, "battery17voltage"=0.0, "battery18voltage"=0.0, "battery19voltage"=0.0, "battery20voltage"=0.0, "battery21voltage"=0.0, "battery22voltage"=0.0, "battery23voltage"=0.0, "battery24voltage"=0.0, "ErrorOutData"={"ErrorCode"=0, "ErrorMessage"=""}}, {"battery1voltage"=3.4816356, "battery2voltage"=3.4830368, "battery3voltage"=3.4783683, "battery4voltage"=3.4823706, "battery5voltage"=3.4844058, "battery6voltage"=0.0, "battery7voltage"=0.0, "battery8voltage"=0.0, "battery9voltage"=0.0, "battery10voltage"=0.0, "battery11voltage"=0.0, "battery12voltage"=0.0, "battery13voltage"=0.0, "battery14voltage"=0.0, "battery15voltage"=0.0, "battery16voltage"=0.0, "battery17voltage"=0.0, "battery18voltage"=0.0, "battery19voltage"=0.0, "battery20voltage"=0.0, "battery21voltage"=0.0, "battery22voltage"=0.0, "battery23voltage"=0.0, "battery24voltage"=0.0, "ErrorOutData"={"ErrorCode"=0, "ErrorMessage"=""}}, {"battery1voltage"=3.4816363, "battery2voltage"=3.4830387, "battery3voltage"=3.478373, "battery4voltage"=3.4823644, "battery5voltage"=3.4844077, "battery6voltage"=0.0, "battery7voltage"=0.0, "battery8voltage"=0.0, "battery9voltage"=0.0, "battery10voltage"=0.0, "battery11voltage"=0.0, "battery12voltage"=0.0, "battery13voltage"=0.0, "battery14voltage"=0.0, "battery15voltage"=0.0, "battery16voltage"=0.0, "battery17voltage"=0.0, "battery18voltage"=0.0, "battery19voltage"=0.0, "battery20voltage"=0.0, "battery21voltage"=0.0, "battery22voltage"=0.0, "battery23voltage"=0.0, "battery24voltage"=0.0, "ErrorOutData"={"ErrorCode"=0, "ErrorMessage"=""}}, {"battery1voltage"=3.4816382, "battery2voltage"=3.4830468, "battery3voltage"=3.478372, "battery4voltage"=3.4823663, "battery5voltage"=3.4844036, "battery6voltage"=0.0, "battery7voltage"=0.0, "battery8voltage"=0.0, "battery9voltage"=0.0, "battery10voltage"=0.0, "battery11voltage"=0.0, "battery12voltage"=0.0, "battery13voltage"=0.0, "battery14voltage"=0.0, "battery15voltage"=0.0, "battery16voltage"=0.0, "battery17voltage"=0.0, "battery18voltage"=0.0, "battery19voltage"=0.0, "battery20voltage"=0.0, "battery21voltage"=0.0, "battery22voltage"=0.0, "battery23voltage"=0.0, "battery24voltage"=0.0, "ErrorOutData"={"ErrorCode"=0, "ErrorMessage"=""}}, {"battery1voltage"=3.4816408, "battery2voltage"=3.4830465, "battery3voltage"=3.478378, "battery4voltage"=3.48237, "battery5voltage"=3.4843988, "battery6voltage"=0.0, "battery7voltage"=0.0, "battery8voltage"=0.0, "battery9voltage"=0.0, "battery10voltage"=0.0, "battery11voltage"=0.0, "battery12voltage"=0.0, "battery13voltage"=0.0, "battery14voltage"=0.0, "battery15voltage"=0.0, "battery16voltage"=0.0, "battery17voltage"=0.0, "battery18voltage"=0.0, "battery19voltage"=0.0, "battery20voltage"=0.0, "battery21voltage"=0.0, "battery22voltage"=0.0, "battery23voltage"=0.0, "battery24voltage"=0.0, "ErrorOutData"={"ErrorCode"=0, "ErrorMessage"=""}}, {"battery1voltage"=3.48164, "battery2voltage"=3.4830382, "battery3voltage"=3.4783747, "battery4voltage"=3.4823658, "battery5voltage"=3.4843998, "battery6voltage"=0.0, "battery7voltage"=0.0, "battery8voltage"=0.0, "battery9voltage"=0.0, "battery10voltage"=0.0, "battery11voltage"=0.0, "battery12voltage"=0.0, "battery13voltage"=0.0, "battery14voltage"=0.0, "battery15voltage"=0.0, "battery16voltage"=0.0, "battery17voltage"=0.0, "battery18voltage"=0.0, "battery19voltage"=0.0, "battery20voltage"=0.0, "battery21voltage"=0.0, "battery22voltage"=0.0, "battery23voltage"=0.0, "battery24voltage"=0.0, "ErrorOutData"={"ErrorCode"=0, "ErrorMessage"=""}}, {"battery1voltage"=3.481639, "battery2voltage"=3.4830444, "battery3voltage"=3.4783697, "battery4voltage"=3.482369, "battery5voltage"=3.4844058, "battery6voltage"=0.0, "battery7voltage"=0.0, "battery8voltage"=0.0, "battery9voltage"=0.0, "battery10voltage"=0.0, "battery11voltage"=0.0, "battery12voltage"=0.0, "battery13voltage"=0.0, "battery14voltage"=0.0, "battery15voltage"=0.0, "battery16voltage"=0.0, "battery17voltage"=0.0, "battery18voltage"=0.0, "battery19voltage"=0.0, "battery20voltage"=0.0, "battery21voltage"=0.0, "battery22voltage"=0.0, "battery23voltage"=0.0, "battery24voltage"=0.0, "ErrorOutData"={"ErrorCode"=0, "ErrorMessage"=""}}, {"battery1voltage"=3.4816341, "battery2voltage"=3.483041, "battery3voltage"=3.4783704, "battery4voltage"=3.4823651, "battery5voltage"=3.4844072, "battery6voltage"=0.0, "battery7voltage"=0.0, "battery8voltage"=0.0, "battery9voltage"=0.0, "battery10voltage"=0.0, "battery11voltage"=0.0, "battery12voltage"=0.0, "battery13voltage"=0.0, "battery14voltage"=0.0, "battery15voltage"=0.0, "battery16voltage"=0.0, "battery17voltage"=0.0, "battery18voltage"=0.0, "battery19voltage"=0.0, "battery20voltage"=0.0, "battery21voltage"=0.0, "battery22voltage"=0.0, "battery23voltage"=0.0, "battery24voltage"=0.0, "ErrorOutData"={"ErrorCode"=0, "ErrorMessage"=""}}, {"battery1voltage"=3.481641, "battery2voltage"=3.4830418, "battery3voltage"=3.4783719, "battery4voltage"=3.482372, "battery5voltage"=3.4844098, "battery6voltage"=0.0, "battery7voltage"=0.0, "battery8voltage"=0.0, "battery9voltage"=0.0, "battery10voltage"=0.0, "battery11voltage"=0.0, "battery12voltage"=0.0, "battery13voltage"=0.0, "battery14voltage"=0.0, "battery15voltage"=0.0, "battery16voltage"=0.0, "battery17voltage"=0.0, "battery18voltage"=0.0, "battery19voltage"=0.0, "battery20voltage"=0.0, "battery21voltage"=0.0, "battery22voltage"=0.0, "battery23voltage"=0.0, "battery24voltage"=0.0, "ErrorOutData"={"ErrorCode"=0, "ErrorMessage"=""}}, {"battery1voltage"=3.4816356, "battery2voltage"=3.4830396, "battery3voltage"=3.478371, "battery4voltage"=3.4823728, "battery5voltage"=3.4844012, "battery6voltage"=0.0, "battery7voltage"=0.0, "battery8voltage"=0.0, "battery9voltage"=0.0, "battery10voltage"=0.0, "battery11voltage"=0.0, "battery12voltage"=0.0, "battery13voltage"=0.0, "battery14voltage"=0.0, "battery15voltage"=0.0, "battery16voltage"=0.0, "battery17voltage"=0.0, "battery18voltage"=0.0, "battery19voltage"=0.0, "battery20voltage"=0.0, "battery21voltage"=0.0, "battery22voltage"=0.0, "battery23voltage"=0.0, "battery24voltage"=0.0, "ErrorOutData"={"ErrorCode"=0, "ErrorMessage"=""}}, {"battery1voltage"=3.4816346, "battery2voltage"=3.483039, "battery3voltage"=3.478373, "battery4voltage"=3.4823637, "battery5voltage"=3.4844048, "battery6voltage"=0.0, "battery7voltage"=0.0, "battery8voltage"=0.0, "battery9voltage"=0.0, "battery10voltage"=0.0, "battery11voltage"=0.0, "battery12voltage"=0.0, "battery13voltage"=0.0, "battery14voltage"=0.0, "battery15voltage"=0.0, "battery16voltage"=0.0, "battery17voltage"=0.0, "battery18voltage"=0.0, "battery19voltage"=0.0, "battery20voltage"=0.0, "battery21voltage"=0.0, "battery22voltage"=0.0, "battery23voltage"=0.0, "battery24voltage"=0.0, "ErrorOutData"={"ErrorCode"=0, "ErrorMessage"=""}}, {"battery1voltage"=3.4816375, "battery2voltage"=3.4830399, "battery3voltage"=3.4783738, "battery4voltage"=3.4823651, "battery5voltage"=3.4844062, "battery6voltage"=0.0, "battery7voltage"=0.0, "battery8voltage"=0.0, "battery9voltage"=0.0, "battery10voltage"=0.0, "battery11voltage"=0.0, "battery12voltage"=0.0, "battery13voltage"=0.0, "battery14voltage"=0.0, "battery15voltage"=0.0, "battery16voltage"=0.0, "battery17voltage"=0.0, "battery18voltage"=0.0, "battery19voltage"=0.0, "battery20voltage"=0.0, "battery21voltage"=0.0, "battery22voltage"=0.0, "battery23voltage"=0.0, "battery24voltage"=0.0, "ErrorOutData"={"ErrorCode"=0, "ErrorMessage"=""}}, {"battery1voltage"=3.4816372, "battery2voltage"=3.4830463, "battery3voltage"=3.478377, "battery4voltage"=3.4823728, "battery5voltage"=3.484404, "battery6voltage"=0.0, "battery7voltage"=0.0, "battery8voltage"=0.0, "battery9voltage"=0.0, "battery10voltage"=0.0, "battery11voltage"=0.0, "battery12voltage"=0.0, "battery13voltage"=0.0, "battery14voltage"=0.0, "battery15voltage"=0.0, "battery16voltage"=0.0, "battery17voltage"=0.0, "battery18voltage"=0.0, "battery19voltage"=0.0, "battery20voltage"=0.0, "battery21voltage"=0.0, "battery22voltage"=0.0, "battery23voltage"=0.0, "battery24voltage"=0.0, "ErrorOutData"={"ErrorCode"=0, "ErrorMessage"=""}}, {"battery1voltage"=3.481637, "battery2voltage"=3.4830413, "battery3voltage"=3.4783728, "battery4voltage"=3.482369, "battery5voltage"=3.484405, "battery6voltage"=0.0, "battery7voltage"=0.0, "battery8voltage"=0.0, "battery9voltage"=0.0, "battery10voltage"=0.0, "battery11voltage"=0.0, "battery12voltage"=0.0, "battery13voltage"=0.0, "battery14voltage"=0.0, "battery15voltage"=0.0, "battery16voltage"=0.0, "battery17voltage"=0.0, "battery18voltage"=0.0, "battery19voltage"=0.0, "battery20voltage"=0.0, "battery21voltage"=0.0, "battery22voltage"=0.0, "battery23voltage"=0.0, "battery24voltage"=0.0, "ErrorOutData"={"ErrorCode"=0, "ErrorMessage"=""}}, {"battery1voltage"=3.4816399, "battery2voltage"=3.4830387, "battery3voltage"=3.4783702, "battery4voltage"=3.4823713, "battery5voltage"=3.4844084, "battery6voltage"=0.0, "battery7voltage"=0.0, "battery8voltage"=0.0, "battery9voltage"=0.0, "battery10voltage"=0.0, "battery11voltage"=0.0, "battery12voltage"=0.0, "battery13voltage"=0.0, "battery14voltage"=0.0, "battery15voltage"=0.0, "battery16voltage"=0.0, "battery17voltage"=0.0, "battery18voltage"=0.0, "battery19voltage"=0.0, "battery20voltage"=0.0, "battery21voltage"=0.0, "battery22voltage"=0.0, "battery23voltage"=0.0, "battery24voltage"=0.0, "ErrorOutData"={"ErrorCode"=0, "ErrorMessage"=""}}, {"battery1voltage"=3.4816375, "battery2voltage"=3.4830422, "battery3voltage"=3.4783688, "battery4voltage"=3.4823675, "battery5voltage"=3.4843993, "battery6voltage"=0.0, "battery7voltage"=0.0, "battery8voltage"=0.0, "battery9voltage"=0.0, "battery10voltage"=0.0, "battery11voltage"=0.0, "battery12voltage"=0.0, "battery13voltage"=0.0, "battery14voltage"=0.0, "battery15voltage"=0.0, "battery16voltage"=0.0, "battery17voltage"=0.0, "battery18voltage"=0.0, "battery19voltage"=0.0, "battery20voltage"=0.0, "battery21voltage"=0.0, "battery22voltage"=0.0, "battery23voltage"=0.0, "battery24voltage"=0.0, "ErrorOutData"={"ErrorCode"=0, "ErrorMessage"=""}}, {"battery1voltage"=3.4816432, "battery2voltage"=3.4830387, "battery3voltage"=3.478373, "battery4voltage"=3.482368, "battery5voltage"=3.484403, "battery6voltage"=0.0, "battery7voltage"=0.0, "battery8voltage"=0.0, "battery9voltage"=0.0, "battery10voltage"=0.0, "battery11voltage"=0.0, "battery12voltage"=0.0, "battery13voltage"=0.0, "battery14voltage"=0.0, "battery15voltage"=0.0, "battery16voltage"=0.0, "battery17voltage"=0.0, "battery18voltage"=0.0, "battery19voltage"=0.0, "battery20voltage"=0.0, "battery21voltage"=0.0, "battery22voltage"=0.0, "battery23voltage"=0.0, "battery24voltage"=0.0, "ErrorOutData"={"ErrorCode"=0, "ErrorMessage"=""}}, {"battery1voltage"=3.4816358, "battery2voltage"=3.483043, "battery3voltage"=3.4783685, "battery4voltage"=3.4823685, "battery5voltage"=3.484403, "battery6voltage"=0.0, "battery7voltage"=0.0, "battery8voltage"=0.0, "battery9voltage"=0.0, "battery10voltage"=0.0, "battery11voltage"=0.0, "battery12voltage"=0.0, "battery13voltage"=0.0, "battery14voltage"=0.0, "battery15voltage"=0.0, "battery16voltage"=0.0, "battery17voltage"=0.0, "battery18voltage"=0.0, "battery19voltage"=0.0, "battery20voltage"=0.0, "battery21voltage"=0.0, "battery22voltage"=0.0, "battery23voltage"=0.0, "battery24voltage"=0.0, "ErrorOutData"={"ErrorCode"=0, "ErrorMessage"=""}}, {"battery1voltage"=3.4816375, "battery2voltage"=3.483041, "battery3voltage"=3.4783714, "battery4voltage"=3.4823701, "battery5voltage"=3.484405, "battery6voltage"=0.0, "battery7voltage"=0.0, "battery8voltage"=0.0, "battery9voltage"=0.0, "battery10voltage"=0.0, "battery11voltage"=0.0, "battery12voltage"=0.0, "battery13voltage"=0.0, "battery14voltage"=0.0, "battery15voltage"=0.0, "battery16voltage"=0.0, "battery17voltage"=0.0, "battery18voltage"=0.0, "battery19voltage"=0.0, "battery20voltage"=0.0, "battery21voltage"=0.0, "battery22voltage"=0.0, "battery23voltage"=0.0, "battery24voltage"=0.0, "ErrorOutData"={"ErrorCode"=0, "ErrorMessage"=""}}, {"battery1voltage"=3.48164, "battery2voltage"=3.4830444, "battery3voltage"=3.4783697, "battery4voltage"=3.4823718, "battery5voltage"=3.4844031, "battery6voltage"=0.0, "battery7voltage"=0.0, "battery8voltage"=0.0, "battery9voltage"=0.0, "battery10voltage"=0.0, "battery11voltage"=0.0, "battery12voltage"=0.0, "battery13voltage"=0.0, "battery14voltage"=0.0, "battery15voltage"=0.0, "battery16voltage"=0.0, "battery17voltage"=0.0, "battery18voltage"=0.0, "battery19voltage"=0.0, "battery20voltage"=0.0, "battery21voltage"=0.0, "battery22voltage"=0.0, "battery23voltage"=0.0, "battery24voltage"=0.0, "ErrorOutData"={"ErrorCode"=0, "ErrorMessage"=""}}, {"battery1voltage"=3.4816394, "battery2voltage"=3.4830453, "battery3voltage"=3.4783723, "battery4voltage"=3.4823713, "battery5voltage"=3.4843984, "battery6voltage"=0.0, "battery7voltage"=0.0, "battery8voltage"=0.0, "battery9voltage"=0.0, "battery10voltage"=0.0, "battery11voltage"=0.0, "battery12voltage"=0.0, "battery13voltage"=0.0, "battery14voltage"=0.0, "battery15voltage"=0.0, "battery16voltage"=0.0, "battery17voltage"=0.0, "battery18voltage"=0.0, "battery19voltage"=0.0, "battery20voltage"=0.0, "battery21voltage"=0.0, "battery22voltage"=0.0, "battery23voltage"=0.0, "battery24voltage"=0.0, "ErrorOutData"={"ErrorCode"=0, "ErrorMessage"=""}}, {"battery1voltage"=3.4816341, "battery2voltage"=3.4830413, "battery3voltage"=3.4783728, "battery4voltage"=3.4823737, "battery5voltage"=3.4844046, "battery6voltage"=0.0, "battery7voltage"=0.0, "battery8voltage"=0.0, "battery9voltage"=0.0, "battery10voltage"=0.0, "battery11voltage"=0.0, "battery12voltage"=0.0, "battery13voltage"=0.0, "battery14voltage"=0.0, "battery15voltage"=0.0, "battery16voltage"=0.0, "battery17voltage"=0.0, "battery18voltage"=0.0, "battery19voltage"=0.0, "battery20voltage"=0.0, "battery21voltage"=0.0, "battery22voltage"=0.0, "battery23voltage"=0.0, "battery24voltage"=0.0, "ErrorOutData"={"ErrorCode"=0, "ErrorMessage"=""}}, {"battery1voltage"=3.4816387, "battery2voltage"=3.4830446, "battery3voltage"=3.4783685, "battery4voltage"=3.482368, "battery5voltage"=3.4844067, "battery6voltage"=0.0, "battery7voltage"=0.0, "battery8voltage"=0.0, "battery9voltage"=0.0, "battery10voltage"=0.0, "battery11voltage"=0.0, "battery12voltage"=0.0, "battery13voltage"=0.0, "battery14voltage"=0.0, "battery15voltage"=0.0, "battery16voltage"=0.0, "battery17voltage"=0.0, "battery18voltage"=0.0, "battery19voltage"=0.0, "battery20voltage"=0.0, "battery21voltage"=0.0, "battery22voltage"=0.0, "battery23voltage"=0.0, "battery24voltage"=0.0, "ErrorOutData"={"ErrorCode"=0, "ErrorMessage"=""}}, {"battery1voltage"=3.4816349, "battery2voltage"=3.48304, "battery3voltage"=3.4783728, "battery4voltage"=3.482367, "battery5voltage"=3.4844062, "battery6voltage"=0.0, "battery7voltage"=0.0, "battery8voltage"=0.0, "battery9voltage"=0.0, "battery10voltage"=0.0, "battery11voltage"=0.0, "battery12voltage"=0.0, "battery13voltage"=0.0, "battery14voltage"=0.0, "battery15voltage"=0.0, "battery16voltage"=0.0, "battery17voltage"=0.0, "battery18voltage"=0.0, "battery19voltage"=0.0, "battery20voltage"=0.0, "battery21voltage"=0.0, "battery22voltage"=0.0, "battery23voltage"=0.0, "battery24voltage"=0.0, "ErrorOutData"={"ErrorCode"=0, "ErrorMessage"=""}}, {"battery1voltage"=3.4816382, "battery2voltage"=3.483041, "battery3voltage"=3.4783733, "battery4voltage"=3.4823716, "battery5voltage"=3.4844053, "battery6voltage"=0.0, "battery7voltage"=0.0, "battery8voltage"=0.0, "battery9voltage"=0.0, "battery10voltage"=0.0, "battery11voltage"=0.0, "battery12voltage"=0.0, "battery13voltage"=0.0, "battery14voltage"=0.0, "battery15voltage"=0.0, "battery16voltage"=0.0, "battery17voltage"=0.0, "battery18voltage"=0.0, "battery19voltage"=0.0, "battery20voltage"=0.0, "battery21voltage"=0.0, "battery22voltage"=0.0, "battery23voltage"=0.0, "battery24voltage"=0.0, "ErrorOutData"={"ErrorCode"=0, "ErrorMessage"=""}}, {"battery1voltage"=3.481638, "battery2voltage"=3.4830427, "battery3voltage"=3.4783704, "battery4voltage"=3.4823666, "battery5voltage"=3.4844048, "battery6voltage"=0.0, "battery7voltage"=0.0, "battery8voltage"=0.0, "battery9voltage"=0.0, "battery10voltage"=0.0, "battery11voltage"=0.0, "battery12voltage"=0.0, "battery13voltage"=0.0, "battery14voltage"=0.0, "battery15voltage"=0.0, "battery16voltage"=0.0, "battery17voltage"=0.0, "battery18voltage"=0.0, "battery19voltage"=0.0, "battery20voltage"=0.0, "battery21voltage"=0.0, "battery22voltage"=0.0, "battery23voltage"=0.0, "battery24voltage"=0.0, "ErrorOutData"={"ErrorCode"=0, "ErrorMessage"=""}}, {"battery1voltage"=3.4816375, "battery2voltage"=3.4830396, "battery3voltage"=3.4783683, "battery4voltage"=3.482369, "battery5voltage"=3.4844077, "battery6voltage"=0.0, "battery7voltage"=0.0, "battery8voltage"=0.0, "battery9voltage"=0.0, "battery10voltage"=0.0, "battery11voltage"=0.0, "battery12voltage"=0.0, "battery13voltage"=0.0, "battery14voltage"=0.0, "battery15voltage"=0.0, "battery16voltage"=0.0, "battery17voltage"=0.0, "battery18voltage"=0.0, "battery19voltage"=0.0, "battery20voltage"=0.0, "battery21voltage"=0.0, "battery22voltage"=0.0, "battery23voltage"=0.0, "battery24voltage"=0.0, "ErrorOutData"={"ErrorCode"=0, "ErrorMessage"=""}}, {"battery1voltage"=3.4816344, "battery2voltage"=3.4830408, "battery3voltage"=3.4783728, "battery4voltage"=3.4823692, "battery5voltage"=3.4844024, "battery6voltage"=0.0, "battery7voltage"=0.0, "battery8voltage"=0.0, "battery9voltage"=0.0, "battery10voltage"=0.0, "battery11voltage"=0.0, "battery12voltage"=0.0, "battery13voltage"=0.0, "battery14voltage"=0.0, "battery15voltage"=0.0, "battery16voltage"=0.0, "battery17voltage"=0.0, "battery18voltage"=0.0, "battery19voltage"=0.0, "battery20voltage"=0.0, "battery21voltage"=0.0, "battery22voltage"=0.0, "battery23voltage"=0.0, "battery24voltage"=0.0, "ErrorOutData"={"ErrorCode"=0, "ErrorMessage"=""}}, {"battery1voltage"=3.4816382, "battery2voltage"=3.483045, "battery3voltage"=3.478367, "battery4voltage"=3.4823682, "battery5voltage"=3.484407, "battery6voltage"=0.0, "battery7voltage"=0.0, "battery8voltage"=0.0, "battery9voltage"=0.0, "battery10voltage"=0.0, "battery11voltage"=0.0, "battery12voltage"=0.0, "battery13voltage"=0.0, "battery14voltage"=0.0, "battery15voltage"=0.0, "battery16voltage"=0.0, "battery17voltage"=0.0, "battery18voltage"=0.0, "battery19voltage"=0.0, "battery20voltage"=0.0, "battery21voltage"=0.0, 
